vi "Set Variant Name.vi"(8 "error in":errorcluster, 10 "Name":string, 11 "Variant_in":variant) -> (0 "error out":errorcluster, 3 "Variant_out":variant)   [LabVIEW 2021, in "DataTypes_CIF_U.lvlib"]
doc: "This will set an attribute of \"Name\" on a variant."
uses:
  DataTypes_CIF_U.lvlib
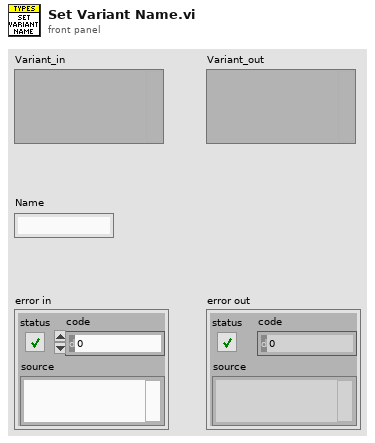
[diagram p1: front panel]
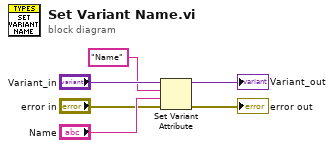
[diagram p0: block diagram]
diagram:
  n1 = Set Variant Attribute(Variant="Variant_in", name="Name", value="Name", error in="error in") -> (Variant out=→"Variant_out":variant, error out=→"error out":errorcluster)  [unwired: 1 out]
